vi "4461.Start.AO.vi"(8 "error in (no error)":errorcluster, 11 "LockinDAQ":refnum<class "LockinDAQ.lvclass">) -> (0 "error out":errorcluster, 3 "LockinDAQ out":refnum<class "LockinDAQ.lvclass">)   [LabVIEW 2016, in "LockinDAQ.lvclass"]
uses:
  LockinDAQ.lvclass
  LockinDAQ.lvclass/LockinDAQ.ctl
  <vilib>/DAQmx/write.llb/DAQmx Write (Analog 1D Wfm NChan NSamp).vi
  <vilib>/DAQmx/miscellaneous.llb/DAQmx Fill In Error Info.vi
panel:
  out "Array":u32[](array[numeric])
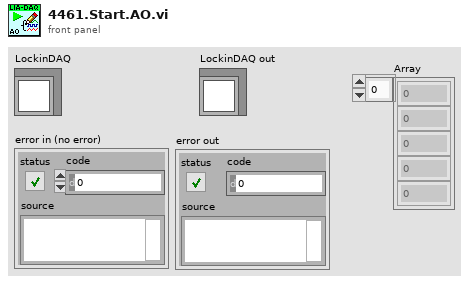
[diagram p1: front panel]
types:
  T1 = typedef "LockinDAQ.lvclass/AO-cluster.ctl" = cluster{"AO Amp (V)":T2, "AO DC (V)":T3, "AO f (Hz)":T4, "AO Phase (°)":T5, "Function":T6, "I+":bool[], "Sweeping":bool[]}
  T2 = typedef "LockinDAQ.lvclass/AO_Amp-array.ctl" = dbl[]
  T3 = typedef "LockinDAQ.lvclass/AO_DC-array.ctl" = dbl[]
  T4 = typedef "LockinDAQ.lvclass/AO_f-array.ctl" = dbl[]
  T5 = typedef "LockinDAQ.lvclass/AO_phi-array.ctl" = dbl[]
  T6 = typedef "LockinDAQ.lvclass/Function-array.ctl" = T7[]
  T7 = typedef "LockinDAQ.lvclass/Function-enum.ctl" = enum16{"Sine", "Triangle", "Square", "Sawtooth"}
  T8 = typedef "LockinDAQ.lvclass/REF-cluster.ctl" = cluster{"REF f (Hz)":T9, "REF phi (°)":T10}
  T9 = typedef "LockinDAQ.lvclass/REF_f-array.ctl" = dbl[]
  T10 = typedef "LockinDAQ.lvclass/REF_phi-array.ctl" = dbl[]
  T11 = typedef "LockinDAQ.lvclass/Sampling.ctl" = cluster{"Fs":dbl, "#s":i32}
  T12 = typedef "LockinDAQ.lvclass/DAQType-enum.ctl" = enum16{"None", "USB 4431", "PXI 446x"}
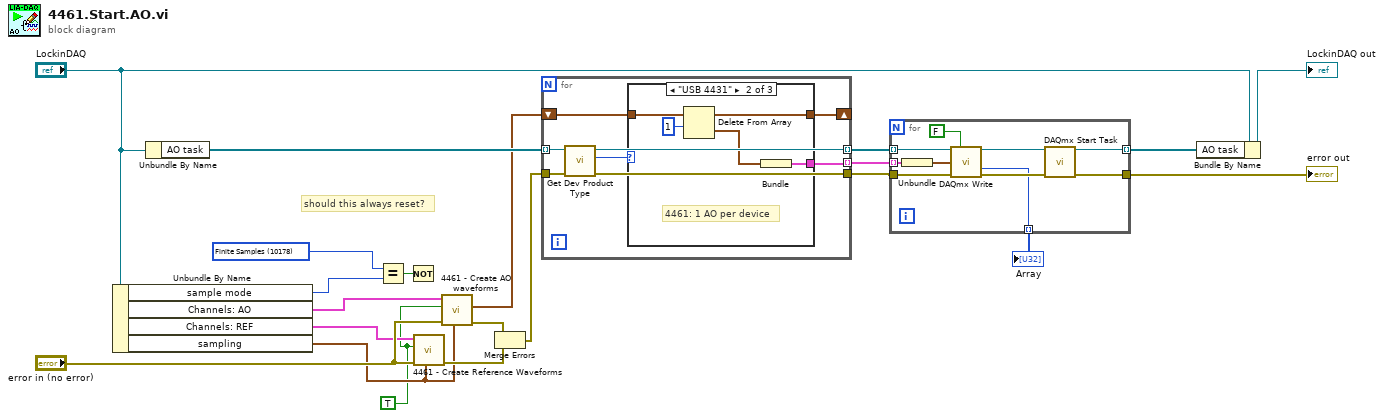
[diagram p0: block diagram]
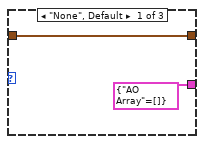
[diagram p2: hidden frame]
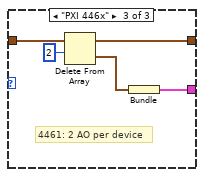
[diagram p3: hidden frame]
diagram:
  w1 = TRUE ("reset signal")
  w15 = 10178 items=["Finite Samples"=10178, "Continuous Samples"=10123] ("sample mode 2")
  # "should this always reset?"
  n1 = Unbundle By Name("LockinDAQ") -> ("sample mode"=w16:i32, "Channels: AO"=w18:T1, "Channels: REF"=w17:T8, "sampling"=w5:T11)
  n2 = Unbundle By Name("LockinDAQ") -> ("AO task"=w10:refnum<k21>[])
  n3 = Equal?(x=w15, y=w16) -> (x = y?=w19:bool)
  n4 = Not(x=w19) -> ()  [unwired: 1 out]
  n5 = call "4461 - Create Reference Waveforms.vi"("sampling"=w5, "error in (no error)"="error in (no error)", "reset signal"=w1, "Lockin"=w17) -> ("error out"=w21:errorcluster)  [unwired: 4 in, 3 out]
  n6 = call "4461 - Create AO waveforms.vi"("sampling"=w5, "error in (no error)"="error in (no error)", "reset signal"=w1, "AO"=w18) -> ("error out"=w4:errorcluster, "AO Array"=w9:waveform(dbl)[])  [unwired: 4 in, 2 out]
  n7 = Merge Errors(w4, w21) -> (w3:errorcluster)
  n8 = for {
    tunnel: w10 -> [w29] mode=indexing
    shift-right: [w27] -> _
    shift-left: w9 -> [w28]
    tunnel: [w26] -> w8 mode=indexing
    tunnel: [w25] -> w7 mode=indexing
    tunnel: w3 -> [w24]
    tunnel: [w23] -> w6
    n9 = call "Get Dev Product Type.vi"("error in (no error)"=w24, "Refnum in"=w29) -> ("error out"=w23:errorcluster, "DAQ Type"=w22:T12, "Refnum out"=w25:refnum<k21>)  [unwired: 6 in, 1 out]
    n10 = case shown="\"USB 4431\"" w22 {
      tunnel: w28 -> [w31 w36 w41]
      tunnel: [w31 w35 w40] -> w27
      tunnel: [cluster{"AO Array":waveform(dbl)[]} {"AO Array"=[]} w33 w37] -> w26
      frame "None", Default {
      }
      frame "USB 4431" {
        # "4461: 1 AO per device"
        n11 = Delete From Array(array=w36, length=1) -> (deleted portion=w32:waveform(dbl)[], array with subset deleted=w35:waveform(dbl)[])  [unwired: 1 in]
        n12 = Bundle("AO Array"=w32) -> (w33:cluster{"AO Array":waveform(dbl)[]})  [unwired: 1 in]
      }
      frame "PXI 446x" {
        # "4461: 2 AO per device"
        n13 = Delete From Array(array=w41, length=2) -> (deleted portion=w38:waveform(dbl)[], array with subset deleted=w40:waveform(dbl)[])  [unwired: 1 in]
        n14 = Bundle("AO Array"=w38) -> (w37:cluster{"AO Array":waveform(dbl)[]})  [unwired: 1 in]
      }
    }
  }
  n15 = for {
    tunnel: w7 -> [w49] mode=indexing
    tunnel: w6 -> [w48]
    tunnel: [w47] -> w11
    tunnel: [w46] -> w12 mode=indexing
    tunnel: w8 -> [w45] mode=indexing
    tunnel: [w42] -> w2 mode=indexing
    n16 = Unbundle(w45) -> ("AO Array"=w44:waveform(dbl)[])
    n17 = call-poly <vilib>:"DAQmx Write.vi"("task/channels in"=w49, "auto start"=FALSE, "data"=w44, "error in"=w48) -> ("task out"=w50:refnum<k21>, "number of samples written per channel"=w42:u32, "error out"=w51:errorcluster)  [unwired: 9 in]
    n18 = call <vilib>:"DAQmx Start Task.vi"("task/channels in"=w50, "error in"=w51) -> ("task out"=w46:refnum<k21>, "error out"=w47:errorcluster)  [unwired: 12 in]
  }
  "error out" <- w11
  "Array" <- w2
  n19 = Bundle By Name(cluster="LockinDAQ", "AO task"=w12) -> (→"LockinDAQ out":refnum<class "LockinDAQ.lvclass">)
